vi "AES Fully Customizable Teeth Generation.vi"(5 "Using Cycle Angle":bool, 6 "FullyCustomTeeth.FirstElement RisingEdge?":bool, 7 "FullyCustomTeeth.Offset":fxp<+/-,61,10>, 8 "Write Timeout?":bool, 9 "FullyCustomTeeth.Next Angle":fxp<+,61,10>, 10 "FullyCustomTeeth.Action":T1, 11 "Crank or Cyle Angle":fxp<+,61,10>) -> (2 "FullyCustomTeeth.Digital Output":bool)   [LabVIEW 2010, in "AES.lvlib" / "AES FPGA.lvlib"]
doc: "This IP generates a digital signal on a digital output line to simulate a singal (usually a cam) that has a varying number of teeth each of varying angle widths. \n\nThe varying number of teeth are provided by passing the angles at which these teeth transitions occur (tooth or gap) to the IP with an input of \"Write CAM Angle\". The first angle provided can be set to a tooth transition (rising edge) or gap transition (falling edge) by specifying the \"First Rising?\" input. \n\nThis IP requires an external angle reference. The reference can be the Cycle Angle (0-720) or the Crank Angle (0-360). Set true on the Using Cycle Angle input if you are using the cycle angle.\n\nOnce all the cam angles have been written to the IP, you should execute the IP in the \"Update CAM Output\" mode so that the IP will begin updating the Cam Digital Output. Note that the \"Write CAM Angle\" mode should only be executed before running in \"Update CAM Output\" mode and that once angles are written they cannot be changed or deleted.\n\nVVT functionality is also provided by passing a Cam Offset to this IP. The Offset can be provided in the range of -512 to 512 in Cycle Angle mode (0-720) or -360 to 360 in Crank Angle mode (0-360)."
uses:
  AES FPGA.lvlib
  FPGA TypeDefs/aes_FullyCustomTeeth ActionEngine Enum.ctl
  <vilib>/rvi/LocalResourceManager/LocalResourceManager.xnode
  <vilib>/rvi/DataTransferAndStorage/Container/Common/niFpgaContainerState.ctl
  <vilib>/rvi/DataTransferAndStorage/Container/Common/niFpgaDataTypeControl.ctl
  <vilib>/rvi/DataTransferAndStorage/Container/Common/niFpgaContainerImplementationControl.ctl
  <vilib>/rvi/DataTransferAndStorage/Container/Common/niFpgaContainerArbitrationOptionsControl.ctl
  <vilib>/rvi/DataTransferAndStorage/Container/Common/niFpgaTransferTypeControl.ctl
  <vilib>/rvi/DataTransferAndStorage/Container/Common/niFpgaContainerInitializationParameters.ctl
  <vilib>/rvi/Memory/Memory_Types/niFpgaMemoryInterfaceConfiguration.ctl
  <vilib>/rvi/FIFO/Fifo_Types/niFpgaFifoControlLogicControl.ctl
  <vilib>/rvi/DataTransferAndStorage/Container/Common/niFpgaContainerMetaDataKey.ctl
  <vilib>/rvi/DataTransferAndStorage/Container/XNode/niFpgaContainer.xnode
  FPGA TypeDefs/aes_FullyCustomTeeth StateMachine Enum.ctl
  <vilib>/rvi/DataTransferAndStorage/Container/Common/niFpgaContainerGetUniqueNameForEmu.vi
  <vilib>/rvi/DataTransferAndStorage/Container/Common/niFpgaContainerSetEmuInfo.vi
  <vilib>/rvi/eio/common/nirviEmuReportErrorAndStop.vi
  <vilib>/rvi/Memory/Memory_Emulation/nirvimemoryEmulationManagerCache_GetValue.vi
  <vilib>/rvi/Memory/Memory_Emulation/nirvimemoryEmulationManagerCache_InsertValue.vi
  <vilib>/Utility/error.llb/Clear Errors.vi
  <vilib>/rvi/Memory/Memory_Emulation/nirvimemoryEmulationManagerCache_SetValue.vi
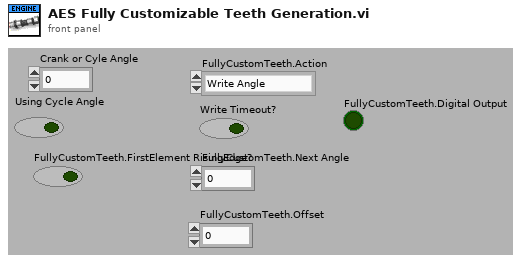
[diagram p1: front panel]
types:
  T1 = typedef "AES.lvlib/AES FPGA.lvlib/aes_FullyCustomTeeth ActionEngine Enum.ctl" = enum16{"Write Angle", "Update Output"}
  T2 = typedef "AES.lvlib/AES FPGA.lvlib/aes_FullyCustomTeeth StateMachine Enum.ctl" = enum16{"Get Next Angle", "Compare Angle", "Wait Until Zero"}
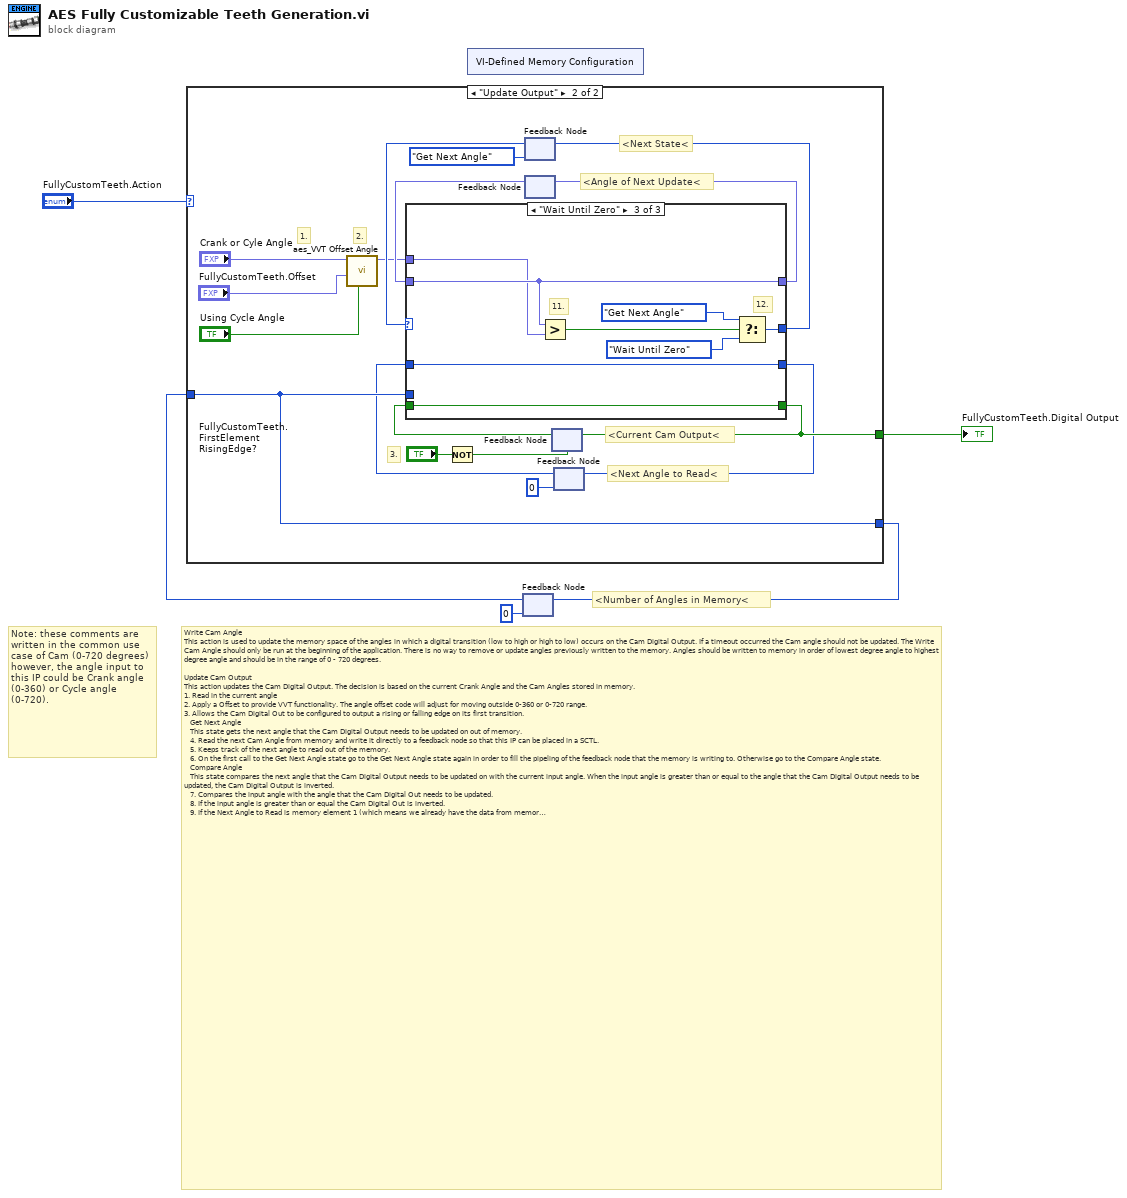
[diagram p0: block diagram]
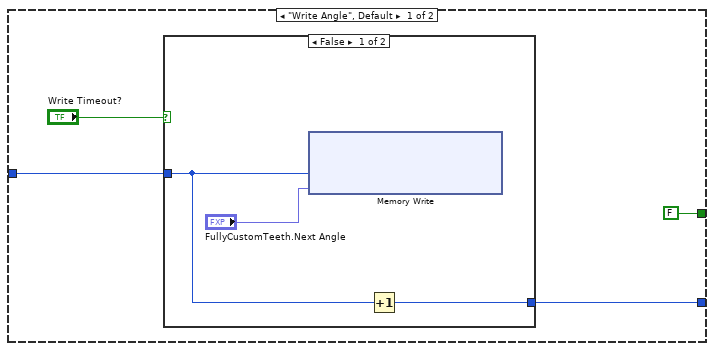
[diagram p2: hidden frame]
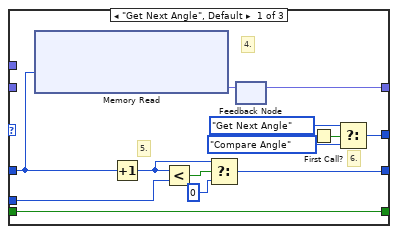
[diagram p4: hidden frame]
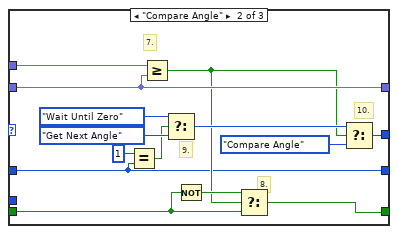
[diagram p5: hidden frame]
diagram:
  # "Note: these comments are written in the common use case of Cam (0-720 degrees) however, the angle input to this IP could be Crank angle (0-360) or Cycle angle (0-720)."
  # "Write Cam Angle\nThis action is used to update the memory space of the angles in which a digital transition (low to high or high to low) occurs on the Cam Digital Output. If a timeout occurred the Cam angle should not be updated. The Write Cam Angle should only be run at the beginning of the application. There is no way to remove or update angles previously written to the memory. Angles should be written to memory in order of lowest degree angle to highest degree angle and should be in the range of 0 - 720 degrees.\n\nUpdate Cam Output\nThis action updates the Cam Digital Output. The decision is based on the current Crank Angle and the Cam Angles stored in memory.\n1. Read in the current angle\n2. Apply a Offset to provide VVT functionality. The angle offset code will adjust for moving outside 0-360 or 0-720 range.\n3. Allows the Cam Digital Out to be configured to output a rising or falling edge on its first transition.\n   Get Next Angle\n   This state gets the next angle that the Cam Digital Output needs to be updated on out of memory.\n   4. Read the next Cam Angle from memory and write it directly to a feedback node so that this IP can be placed in a SCTL.\n   5. Keeps track of the next angle to read out of the memory.\n   6. On the first call to the Get Next Angle state go to the Get Next Angle state again in order to fill the pipeling of the feedback node that the memory is writing to. Otherwise go to the Compare Angle state.\n   Compare Angle\n   This state compares the next angle that the Cam Digital Output needs to be updated on with the current input angle. When the input angle is greater than or equal to the angle that the Cam Digital Output needs to be updated, the Cam Digital Output is inverted.\n   7. Compares the input angle with the angle that the Cam Digital Out needs to be updated.\n   8. If the input angle is greater than or equal the Cam Digital Out is inverted.\n   9. If the Next Angle to Read is memory element 1 (which means we already have the data from memory element 0 ready) and Cam Digital Out is updated, we go to the \"Wait Until Zero\" state to wait until the input Angle rolls back to 0. This keeps our Cam Digital Output from quickly toggling until our input Angle rolls over. If memory element is not 1, we go to \"Get Next Angle\" state if our Cam Digital Out is updated.\n   10. If our Cam Digital Out is not updated we stay in our \"Compare Angle\" state, otherwise we go to \"Get Next Angle\" or \"Wait Until Zero\" depending on step 8.\n   Wait Until Zero \n   Since Cam angles are required to be written to memory from lowest degree angle to highest degree angle, this state is used when we roll back to the first angle stored in memory. This state keeps our Cam Digital Out from incorrectly being updated as we wait for our input Angle to roll back to 0 degrees.\n   11. Compare our input angle with our previously update Cam Digital Out angle. Keep in mind that this Cam Digital Out angle is the highest degree angle stored in our memory.\n   12. When our input angle becomes less than our highest degree Cam angle stored in memory we go to \"Get Next Angle\", otherwise we stay in \"Wait Until Zero\" state."
  # "<Number of Angles in Memory<"
  n1 = xnode "VI-Defined Memory Configuration"() -> ()  [unwired: 1 out]
  n2 = feedback #1(u8 0 ("CAM.Num Angles")) -> (w3:u8)
  n3 = case shown="\"Update Output\"" "FullyCustomTeeth.Action" {
    tunnel: w3 -> [w8 w154]
    tunnel: [FALSE w155] -> w5
    tunnel: [w9 w154] -> w1
    frame "Write Angle", Default {
      n4 = case shown="False" "Write Timeout?" {
        tunnel: [w11 w138] -> w9
        tunnel: w8 -> [w10 w138]
        frame False {
          n5 = xnode ("Memory Write")("Address"=w10, "Data"="FullyCustomTeeth.Next Angle") -> ()  [unwired: 1 in, 1 out]
          n6 = Increment(x=w10) -> (x+1=w11:u8)
        }
        frame True {
        }
      }
    }
    frame "Update Output" {
      # "2."
      # "3."
      # "1."
      # "<Angle of Next Update<"
      # "<Next Angle to Read<"
      # "<Current Cam Output<"
      # "<Next State<"
      n7 = call "aes_VVT Offset Angle.vi"("Using Cycle Angle"="Using Cycle Angle", "Cam.Offset"="FullyCustomTeeth.Offset", "Crank or Cyle Angle"="Crank or Cyle Angle") -> ("Crank.Adjusted Offset Angle"=w142:fxp<+,61,10>)  [unwired: 8 in]
      n8 = Not(x="FullyCustomTeeth.FirstElement RisingEdge?") -> (.not. x?=w153:bool)
      n9 = feedback #2(aes_FullyCustomTeeth_StateMachine_Enum."Get Next Angle" ("Crank Angle Enum")) -> (w148:T2)
      n10 = feedback #3() -> (w146:fxp<+,61,10>)  [unwired: 1 out]
      n11 = feedback #4(w153) -> (w149:bool)
      n12 = feedback #5(u8 0 ("index")) -> (w143:u8)
      n13 = case shown="\"Wait Until Zero\"" w148 {
        tunnel: w143 -> [w168 w297 w313]
        tunnel: [w164 w297 w313] -> w144
        tunnel: [w156 w305 w316] -> w145
        tunnel: w146 -> [_ w305 w316]
        tunnel: [w157 w302 w315] -> w147
        tunnel: [w162 w306 w312] -> w155
        tunnel: w149 -> [w162 w307 w312]
        tunnel: w142 -> [_ w295 w309]
        tunnel: w154 -> [w158 _ _]
        frame "Get Next Angle", Default {
          # "6."
          # "5."
          # "4."
          n14 = xnode ("Memory Read")("Address"=w168) -> ("Data"=w163:fxp<+,61,10>)  [unwired: 1 in, 1 out]
          n15 = Increment(x=w168) -> (x+1=w166:u8)
          n16 = Less?(x=w166, y=w158) -> (x < y?=w167:bool)
          n17 = Select(t=w166, s=w167, f=u8 0) -> (s? t:f=w164:u8)
          n18 = feedback-in #6(w163) -> ()
          n19 = feedback #6() -> (w156:fxp<+,61,10>)  [unwired: 1 out]
          n20 = First Call?() -> (First Call?: T/F=w161:bool)
          n21 = Select(t=aes_FullyCustomTeeth_StateMachine_Enum."Get Next Angle" ("Crank Angle Enum"), s=w161, f=aes_FullyCustomTeeth_StateMachine_Enum."Compare Angle" ("Crank Angle Enum")) -> (s? t:f=w157:T2)
        }
        frame "Compare Angle" {
          # "10."
          # "9."
          # "8."
          # "7."
          n22 = Equal?(x=u8 1, y=w297) -> (x = y?=w298:bool)
          n23 = Greater Or Equal?(x=w295, y=w305) -> (x >= y?=w303:bool)
          n24 = Select(t=aes_FullyCustomTeeth_StateMachine_Enum."Wait Until Zero" ("Crank Angle Enum"), s=w298, f=aes_FullyCustomTeeth_StateMachine_Enum."Get Next Angle" ("Crank Angle Enum")) -> (s? t:f=w304:T2)
          n25 = Not(x=w307) -> (.not. x?=w308:bool)
          n26 = Select(t=w308, s=w303, f=w307) -> (s? t:f=w306:bool)
          n27 = Select(t=w304, s=w303, f=aes_FullyCustomTeeth_StateMachine_Enum."Compare Angle" ("Crank Angle Enum")) -> (s? t:f=w302:T2)
        }
        frame "Wait Until Zero" {
          # "12."
          # "11."
          n28 = Greater?(x=w316, y=w309) -> (0:w314:bool)
          n29 = Select(t=aes_FullyCustomTeeth_StateMachine_Enum."Get Next Angle" ("Crank Angle Enum"), s=w314, f=aes_FullyCustomTeeth_StateMachine_Enum."Wait Until Zero" ("Crank Angle Enum")) -> (s? t:f=w315:T2)
        }
      }
      n30 = feedback-in #2(w147) -> ()
      n31 = feedback-in #3(w145) -> ()
      n32 = feedback-in #4(w155) -> ()
      n33 = feedback-in #5(w144) -> ()
    }
  }
  "FullyCustomTeeth.Digital Output" <- w5
  n34 = feedback-in #1(w1) -> ()
